vi "SSL Context.vi"() -> ()   [LabVIEW 2013, in "suite SSL Client.lvclass"]
uses:
  suite SSL Client.lvclass
  SSL_Lib/SSL-Context/SSL-Context.lvclass
panel:
  in  "SSL-Context":refnum<class "SSL-Context.lvclass">
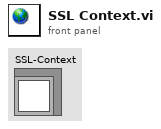
[diagram p1: front panel]
diagram:
